vi "Stop Target Actor.vi"(8 "error in":errorcluster, 11 "MSS Target Actor in":refnum<class "MSS Target Actor.lvclass">) -> (0 "error out":errorcluster, 3 "MSS Target Actor out":refnum<class "MSS Target Actor.lvclass">)   [LabVIEW 2024, in "MSS Target Actor.lvlib" / "MSS Target Actor.lvclass"]
uses:
  MSS Target Actor.lvclass
  MSS Target Actor.lvclass/MSS Target Actor.ctl
  <vilib>/ActorFramework/Actor/Actor.lvclass
  <vilib>/ActorFramework/Stop Msg/Stop Msg.lvclass
  C:/Program Files/National Instruments/LabVIEW 2024/vi.lib/ActorFramework/Actor/Actor.lvclass
  D:/git/HAL/HAL/MSS Target Actor/MSS Target Actor/MSS Target Actor.lvclass
  D:/git/HAL/HAL/MSS Target Actor/IMSS Target Actor/IMSS Target Actor.lvclass
  C:/Program Files/National Instruments/LabVIEW 2024/vi.lib/ni/Actors/Network Endpoint Actors/Nested Endpoint Caller/Nested Endpoint Caller/Nested Endpoint Caller.lvclass
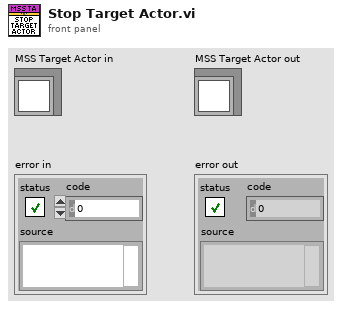
[diagram p1: front panel]
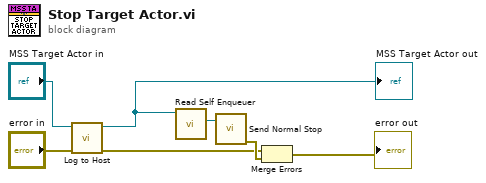
[diagram p0: block diagram]
diagram:
  n1 = call "Log to Host.vi"("error in"="error in", "MSS Target Actor in"="MSS Target Actor in") -> ("error out"=w1:errorcluster, "MSS Target Actor out"=w2:refnum<class "MSS Target Actor.lvclass">)  [unwired: 8 in]
  "MSS Target Actor out" <- w2
  n2 = call <vilib>:"Read Self Enqueuer.vi"("Actor"=w2) -> ("Self Enqueuer"=w5:refnum<class "Message Enqueuer.lvclass">)  [unwired: 10 in]
  n3 = call <vilib>:"Send Normal Stop.vi"("Message Enqueuer"=w5) -> ("error out"=w3:errorcluster)  [unwired: 10 in]
  n4 = Merge Errors(w1, w3) -> (→"error out":errorcluster)
